vi "Teleop.vi"(10 "Match Info":T1={"Autonomous Elapsed Seconds"=0.0, "TeleOp Elapsed Seconds"=0.0, "Disabled Elapsed Seconds"=0.0, "Visited Autonomous"=FALSE, "Visited TeleOp"=FALSE, "Visited Disabled"=FALSE, "Autonomous Settings"={"Autonomous Style"=enum."Independent", "VI Refnum"=refnum}}, 11 "Call Context":T2) -> ()   [LabVIEW 2015]
doc: "This VI is called for each TeleOp packet received from the DS where the robot is not disabled. It is often used to read from the joysticks and update I/O or to update setpoints for timed control loops. It should complete and return within 20 milliseconds or it may miss DS packets."
uses:
  <vilib>/Rock Robotics/WPI/DriverStation/WPI_DriverStationDerivedRobotMode.ctl
  <vilib>/Rock Robotics/WPI/DriverStation/WPI_DriverStationMatch Info.ctl
  <vilib>/Rock Robotics/WPI/RobotDrive/WPI_RobotDriveGetSetRefNum.vi
  Robot Global Data.vi
  <vilib>/Rock Robotics/WPI/Joystick/WPI_JoystickGetSetRefNum.vi
panel:
  out "Numeric 1":dbl(slide) scale=0.0..100.0
  out "Boolean 2":bool
  out "Boolean 1":bool
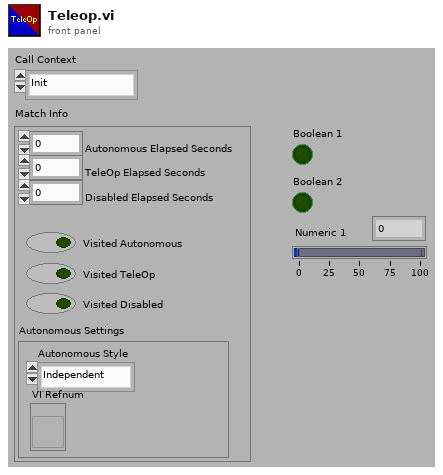
[diagram p1: front panel]
types:
  T1 = typedef "WPI_DriverStationMatch Info.ctl" = cluster{"Autonomous Elapsed Seconds":dbl, "TeleOp Elapsed Seconds":dbl, "Disabled Elapsed Seconds":dbl, "Visited Autonomous":bool, "Visited TeleOp":bool, "Visited Disabled":bool, "Autonomous Settings":cluster{"Autonomous Style":enum16{"Iterative", "Independent"}, "VI Refnum":refnum<vi>}}
  T2 = typedef "WPI_DriverStationDerivedRobotMode.ctl" = enum16{"Init", "Execute", "Stop"}
  T3 = typedef "WPI_JoystickDevRef.ctl" = cluster{"Device":T4}
  T4 = typedef "WPI_JoystickDeviceEnum.ctl" = enum16{"USB 0", "USB 1", "USB 2", "USB 3", "USB 4", "USB 5"}
  T5 = cluster{"Button 1":bool, "Button 2":bool, "Button 3":bool, "Button 4":bool, "Button 5":bool, "Button 6":bool, "Button 7":bool, "Button 8":bool, "Button 9":bool, "Button 10":bool, "Button 11":bool, "Button 12":bool}
  T6 = cluster{"axis 1 (x)":dbl, "axis 2 (y)":dbl, "axis 3 (throttle)":dbl, "axis 4":dbl, "axis 5":dbl, "axis 6":dbl}
  T7 = typedef "WPI_RobotDriveDevRef.ctl" = cluster{"DevStatus":errorcluster, "Motors[]":T8[], "Square Inputs":bool, "Max Output":dbl}
  T8 = typedef "WPI_MotorControlDeviceRef.ctl" = cluster{"DeviceStatus":errorcluster, "Type":enum16{"PWM", "CAN"}, "PWM":cluster{"Digital Module":T9, "PWM Channel":T10, "DeadBand":T11}, "CAN":cluster{"Device Number":u8, "Control Mode":T12, "Semaphore":T13, "Max Vout":dbl}, "Invert":bool, "TransformRef":T14, "InvTransformRef":T14}
  T9 = typedef "FPGA_TypedefDigitalModule.ctl" = enum16{"Digital Module 1", "Digital Module 2"}
  T10 = typedef "FPGA_DIOPWMChannel.ctl" = enum8{"PWM 1", "PWM 2", "PWM 3", "PWM 4", "PWM 5", "PWM 6", "PWM 7", "PWM 8", "PWM 9", "PWM 10", "Invalid"}
  T11 = typedef "WPI_PWMDeadband.ctl" = cluster{"Name":string, "maxPositivePwm":i32, "minPositivePwm":i32, "centerPwm":i32, "maxNegativePwm":i32, "minNegativePwm":i32, "angularRange":u16}
  T12 = typedef "WPI_CANJaguar_ControlMode.ctl" = enum8{"Percent VBus", "Current", "Speed", "Position", "Voltage"}
  T13 = typedef "Semaphore RefNum" = refnum<k1>
  T14 = typedef "WPI_PWMTransform_ConPane.ctl" = refnum<vi>
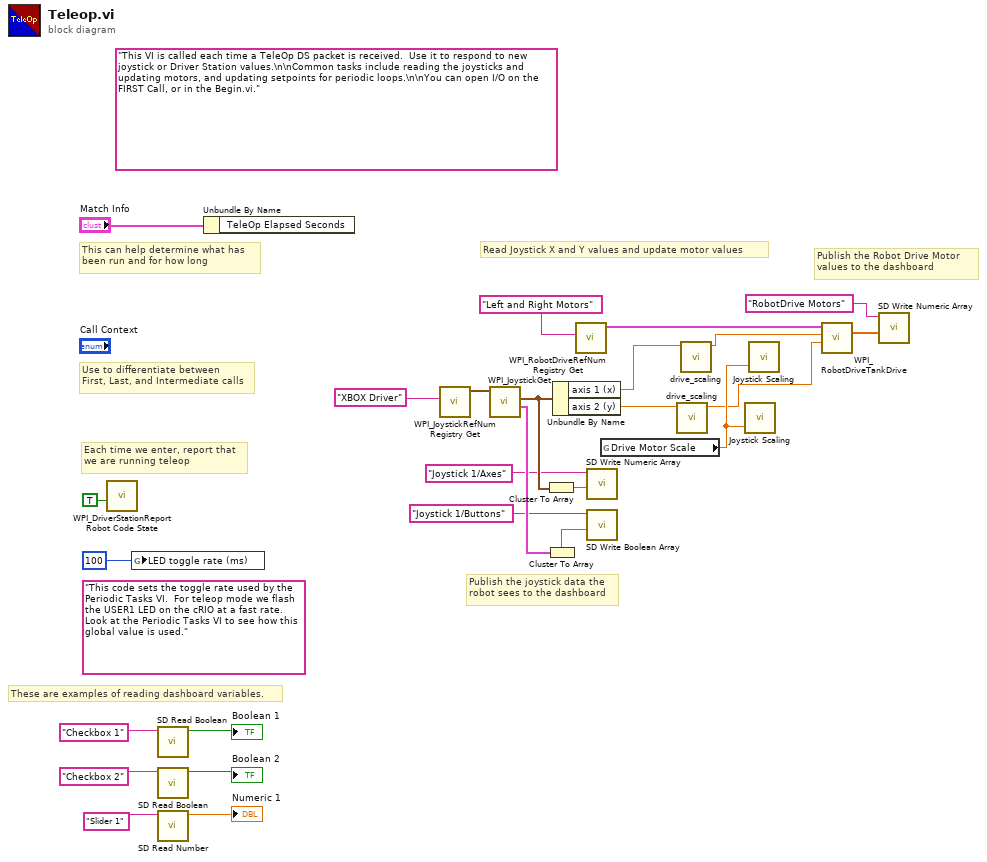
[diagram p0: block diagram]
diagram:
  (unwired) "This code sets the toggle rate used by the Periodic Tasks VI.  For teleop mode we flash the USER1 LED on the cRIO at a fast rate.  Look at the Periodic Tasks VI to see how this global value is used."
  (unwired) "This VI is called each time a TeleOp DS packet is received.  Use it to respond to new joystick or Driver Station values.\n\nCommon tasks include reading the joysticks and updating motors, and updating setpoints for periodic loops.\n\nYou can open I/O on the FIRST Call, or in the Begin.vi."
  # "Publish the Robot Drive Motor\nvalues to the dashboard"
  # "These are examples of reading dashboard variables."
  # "Publish the joystick data the\nrobot sees to the dashboard"
  # "Each time we enter, report that\nwe are running teleop"
  # "Use to differentiate between\nFirst, Last, and Intermediate calls"
  # "This can help determine what has\nbeen run and for how long"
  # "Read Joystick X and Y values and update motor values"
  n1 = call <vilib>:"WPI_DriverStationReport Robot Code State.vi"("TeleOp"=TRUE ("Autonomous")) -> ()  [unwired: 10 in, 1 out]
  n2 = global write "Robot Global Data.vi" "LED toggle rate (ms)"(u32 100 ("LED ms toggle rate")) -> ()
  n3 = call <vilib>:"SD Read Boolean.vi"("Name"="Checkbox 1" ("refnum name")) -> ("Boolean"=→"Boolean 1":bool)  [unwired: 8 in, 2 out]
  n4 = call <vilib>:"SD Read Boolean.vi"("Name"="Checkbox 2" ("refnum name")) -> ("Boolean"=→"Boolean 2":bool)  [unwired: 8 in, 2 out]
  n5 = call <vilib>:"SD Read Number.vi"("Name"="Slider 1" ("refnum name")) -> ("Numeric"=→"Numeric 1":dbl)  [unwired: 8 in, 2 out]
  n6 = Unbundle By Name("Match Info") -> ()  [unwired: 1 out]
  n7 = call <vilib>:"WPI_JoystickRefNum Registry Get.vi"("refnum name"="XBOX Driver") -> ("JoystickDevRef"=w23:T3)  [unwired: 1 in, 9 out]
  n8 = call <vilib>:"WPI_JoystickGet.vi"("JoystickDevRef"=w23) -> ("Buttons"=w20:T5, "Axes"=w17:T6)  [unwired: 1 in, 4 out]
  n9 = Cluster To Array(cluster=w17) -> (array=w16:dbl[])
  n10 = Cluster To Array(cluster=w20) -> (array=w19:bool[])
  n11 = Unbundle By Name(w17) -> ("axis 1 (x)"=w6:dbl, "axis 2 (y)"=w5:dbl)
  n12 = call <vilib>:"WPI_RobotDriveRefNum Registry Get.vi"("refnum name"="Left and Right Motors") -> ("RobotDriveDevRef"=w24:T7)  [unwired: 1 in, 9 out]
  n13 = call <vilib>:"SD Write Numeric Array.vi"("Numeric Array"=w16, "Name"="Joystick 1/Axes") -> ()  [unwired: 8 in, 2 out]
  n14 = call <vilib>:"SD Write Boolean Array.vi"("Boolean Array"=w19, "Name"="Joystick 1/Buttons") -> ()  [unwired: 8 in, 2 out]
  n15 = global read "Robot Global Data.vi" "Drive Motor Scale"() -> (w4:dbl)
  n16 = call "drive_scaling.vi"("In"=w5) -> ("Out"=w2:dbl)  [unwired: 10 in]
  n17 = call "drive_scaling.vi"("In"=w6) -> ("Out"=w1:dbl)  [unwired: 10 in]
  n18 = call "Joystick Scaling.vi"("Scale (%)"=w4) -> ()  [unwired: 2 in, 1 out]
  n19 = call "Joystick Scaling.vi"("Scale (%)"=w4) -> ()  [unwired: 2 in, 1 out]
  n20 = call <vilib>:"WPI_RobotDriveTankDrive.vi"("Right axis value"=w2, "Left axis value"=w1, "RobotDriveDevRef"=w24) -> ("Motor Values"=w13:dbl[])  [unwired: 6 in, 2 out]
  n21 = call <vilib>:"SD Write Numeric Array.vi"("Numeric Array"=w13, "Name"="RobotDrive Motors") -> ()  [unwired: 8 in, 2 out]
